vi "Replace Fixed Parameters.vi"(6 "Fit Model":T2, 8 "Error In":errorcluster, 9 "Fixed Parameter Values (w sigma)":dbl[](array[numeric]), 10 "Fixed Parameter Names":T1[](array[typedef]), 11 "All Guess Parameters in (w tau)":dbl[](array[numeric])) -> (0 "Error Out":errorcluster, 1 "Model Parameter List":T1[](array[typedef]), 2 "Guess Fitted Parameters (w sigma)":dbl[](array[numeric]), 3 "All Guess Parameters out (w sigma)":dbl[](array[numeric]), 4 "All Guess Parameters (w tau)":dbl[](array[numeric]))   [LabVIEW 2021, in "Fits.lvlib"]
doc: "This VI assumes that <B>All Parameters in</B> involve tau, and <B>Fixed Parameters</B> involve sigma = sqrt(tau).\n\nIt returns <B>All Parameters out</B> and <B>Fitted Parameters</B> involving sigma = sqrt(tau).\n\nHowever, <B>Guess Parameters</B> involve tau."
uses:
  Fits.lvlib
  IRF(X)PSED/Decay Fit Parameters In List.ctl
  Decay Model.ctl
  <vilib>/Utility/error.llb/Error Cluster From Error Code.vi
  <vilib>/ErrorRing/Error Ring.xnode
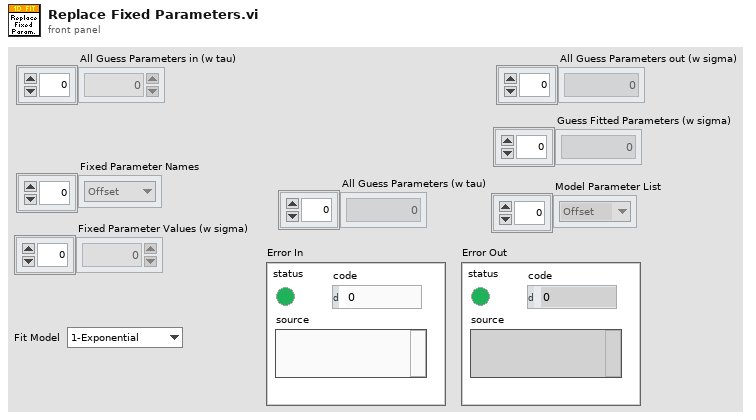
[diagram p1: front panel]
types:
  T1 = typedef "Fits.lvlib/Decay Fit Parameters In List.ctl" = enum16{"Offset", "Baseline", "A_1", "tau_1", "A_2", "tau_2"}
  T2 = typedef "Fits.lvlib/Decay Model.ctl" = enum16{"1-Exponential", "2-Exponentials"}
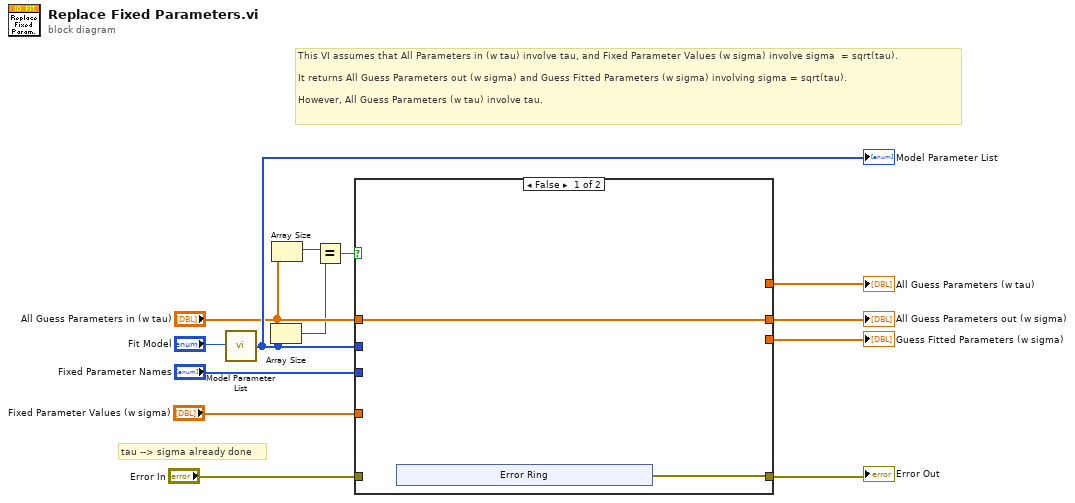
[diagram p0: block diagram]
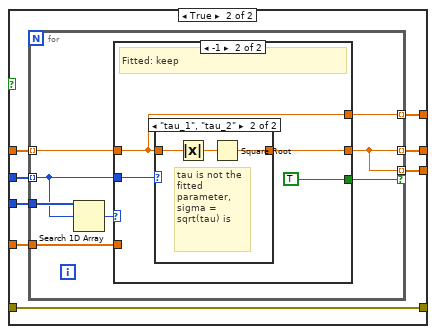
[diagram p2: hidden frame]
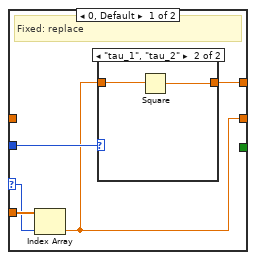
[diagram p3: hidden frame]
diagram:
  # "This VI assumes that All Parameters in (w tau) involve tau, and Fixed Parameter Values (w sigma) involve sigma  = sqrt(tau).\n\nIt returns All Guess Parameters out (w sigma) and Guess Fitted Parameters (w sigma) involving sigma = sqrt(tau).\n\nHowever, All Guess Parameters (w tau) involve tau."
  # "tau --> sigma already done"
  n1 = call "Model Parameter List.vi"("Fit Model"="Fit Model") -> ("Model Parameter List"=w9:T1[])
  "Model Parameter List" <- w9
  n2 = Array Size(array=w9) -> (size(s)=w6:i32)
  n3 = Array Size(array="All Guess Parameters in (w tau)") -> (size(s)=w7:i32)
  n4 = Equal?(x=w7, y=w6) -> (x = y?=w5:bool)
  n5 = case shown="False" w5 {
    tunnel: "Fixed Parameter Names" -> [_ w27]
    tunnel: "Fixed Parameter Values (w sigma)" -> [_ w26]
    tunnel: [w15 w25] -> w10
    tunnel: w9 -> [_ w24]
    tunnel: "All Guess Parameters in (w tau)" -> [w15 w23]
    tunnel: "Error In" -> [_ w22]
    tunnel: [w14 w22] -> w3
    tunnel: [_ w21] -> w2
    tunnel: [_ w20] -> w1
    frame False {
      n6 = xnode "Error Ring"() -> ("error out"=w14:errorcluster)
    }
    frame True {
      n7 = for {
        tunnel: w23 -> [w29] mode=indexing
        tunnel: w24 -> [w31] mode=indexing
        tunnel: w27 -> [w35]
        tunnel: w26 -> [w33]
        tunnel: [w28] -> w25 mode=indexing
        tunnel: [w28] -> w21 mode=indexing if=w32
        tunnel: [w30] -> w20 mode=indexing
        n8 = Search 1D Array(1D array=w35, element=w31) -> (index of element=w34:i32)  [unwired: 1 in]
        n9 = case shown="-1" w34 {
          selector: w34 -> [w39 _]
          tunnel: w33 -> [w40 _]
          tunnel: w29 -> [_ w44]
          tunnel: [w37 w45] -> w28
          tunnel: [_ TRUE] -> w32
          tunnel: w31 -> [w38 w46]
          tunnel: [w36 w44] -> w30
          frame 0, Default {
            # "Fixed: replace"
            n10 = Index Array(array=w40, index=w39) -> (element=w37:dbl)
            n11 = case shown="\"tau_1\", \"tau_2\"" w38 {
              tunnel: w37 -> [w41 w43]
              tunnel: [w41 w42] -> w36
              frame "Offset", Default {
              }
              frame "tau_1", "tau_2" {
                n12 = Square(x=w43) -> (x^2=w42:dbl)
              }
            }
          }
          frame -1 {
            # "Fitted: keep"
            n13 = case shown="\"tau_1\", \"tau_2\"" w46 {
              tunnel: w44 -> [w48 w51]
              tunnel: [w48 w49] -> w45
              frame "Offset", Default {
              }
              frame "tau_1", "tau_2" {
                # "tau is not the fitted parameter, sigma = sqrt(tau) is"
                n14 = Absolute Value(x=w51) -> (abs(x)=w50:dbl)
                n15 = Square Root(x=w50) -> (sqrt(x)=w49:dbl)
              }
            }
          }
        }
      }
    }
  }
  "All Guess Parameters out (w sigma)" <- w10
  "Error Out" <- w3
  "Guess Fitted Parameters (w sigma)" <- w2
  "All Guess Parameters (w tau)" <- w1
